vi "Begin.vi"(8 "error in":errorcluster) -> (0 "error out":errorcluster)   [LabVIEW 2017]
doc: "Called before other user functions, this VI is expected to open initial I/O refnums, load in file data, and do all program initialization. Notice that the <B>error out</B> terminal is simply used for data flow. Wiring it to other structures or subVIs ensures that this VI runs first."
uses:
  <vilib>/Rock Robotics/WPI/DriverStation/WPI_DriverStationRobotMode2.ctl
  <vilib>/Rock Robotics/WPI/Joystick/WPI_JoystickDeviceEnum.ctl
  <vilib>/Rock Robotics/SystemInterfaces/DIO/FPGA_DIOPWMChannel.ctl
  <vilib>/Rock Robotics/WPI/Solenoid/WPI_SolenoidChannel.ctl
  <vilib>/Rock Robotics/WPI/ThirdParty/Cross The Road Electronics/Phoenix-LabVIEW/Motor Controller/Controls/CTRE_Phoenix_MotorControl_ControlMode.ctl
  <vilib>/Rock Robotics/WPI/SafetyOutput/WPI_SafetyOutputConfigMenu.ctl
  <vilib>/Rock Robotics/WPI/ThirdParty/Cross The Road Electronics/Phoenix-LabVIEW/Motor Controller/Controls/CTRE_Phoenix_MotorControl_LimitSwitchSource_Local.ctl
  <vilib>/Rock Robotics/WPI/ThirdParty/Cross The Road Electronics/Phoenix-LabVIEW/Motor Controller/Controls/CTRE_Phoenix_MotorControl_LimitSwitchNormal.ctl
  Robot Global Data.vi
  <vilib>/Rock Robotics/Network Tables/NT Write String Array.vi
  <vilib>/Rock Robotics/Network Tables/NT Write String.vi
  5492_OrientationButtonPress.vi
  5492_DriveOrientation.vi
  5492_SpitButton.vi
  5492_LiftButtons.vi
  5492_DriveRamp.vi
  <vilib>/Rock Robotics/WPI/Solenoid/WPI_SolenoidOpenDouble.vi
  5492_SlowButton.vi
  5492_InitialYaw.vi
  5492_CollectButtons.vi
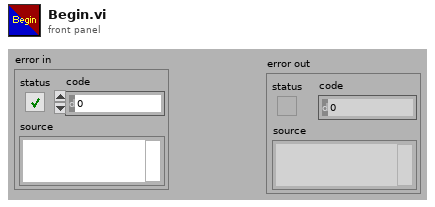
[diagram p1: front panel]
types:
  T1 = typedef "WPI_SafetyOutputConfigMenu.ctl" = enum16{"Enable", "Disable"}
  T2 = typedef "FPGA_DIOPWMChannel.ctl" = enum8{"PWM 0", "PWM 1", "PWM 2", "PWM 3", "PWM 4", "PWM 5", "PWM 6", "PWM 7", "PWM 8", "PWM 9", "PWM MXP 0", "PWM MXP 1", "PWM MXP 2", "PWM MXP 3", "PWM MXP 4", "PWM MXP 5", "PWM MXP 6", "PWM MXP 7", "PWM MXP 8", "PWM MXP 9", "Invalid"}
  T3 = typedef "CTRE_Phoenix_MotorControl_ControlMode.ctl" = u16
  T4 = typedef "CTRE_Phoenix_MotorControl_LimitSwitchNormal.ctl" = enum16{"Normally Open", "Normally Closed", "Disabled"}
  T5 = typedef "CTRE_Phoenix_MotorControl_LimitSwitchSource_Local.ctl" = enum16{"Feedback Connector", "Remote Talon SRX", "Remote CANifier", "Deactivated"}
  T6 = typedef "WPI_SolenoidChannel.ctl" = enum8{"Solenoid 0", "Solenoid 1", "Solenoid 2", "Solenoid 3", "Solenoid 4", "Solenoid 5", "Solenoid 6", "Solenoid 7", "Invalid"}
  T7 = typedef "WPI_JoystickDeviceEnum.ctl" = enum16{"USB 0", "USB 1", "USB 2", "USB 3", "USB 4", "USB 5"}
  T8 = typedef "WPI_DriverStationRobotMode2.ctl" = enum16{"Autonomous Disabled", "Autonomous Enabled", "Teleop Disabled", "Teleop Enabled", "Disconnected", "Finish", "Test Disabled", "Test Enabled", "Emergency Stopped"}
  T9 = typedef "WPI_JoystickDevRef.ctl" = cluster{"Device":T7}
  T10 = typedef "WPI_RobotDriveDevRef.ctl" = cluster{"DevStatus":errorcluster, "Motors[]":T11[], "Square Inputs":bool, "Max Output":dbl}
  T11 = typedef "WPI_MotorControlDeviceRef.ctl" = cluster{"DeviceStatus":errorcluster, "Type":T12, "PWM":cluster{"PWM Channel":T2, "DeadBand":T13}, "CAN":cluster{"Device Number":u8, "SetOutput VI Ref":variant, "GetOutput VI Ref":variant, "Enable VI Ref":variant, "Disable VI Ref":variant, "Data":variant}, "Invert":bool, "DIO PWM":cluster{"PWM \"Enable\" Channel":T2, "DIOChannel":T14, "PWM Rate":dbl}}
  T12 = typedef "WPI_MotorControlType.ctl" = enum16{"PWM", "CAN", "DIO PWM"}
  T13 = typedef "WPI_PWMDeadband.ctl" = cluster{"Name":string, "maxPositivePwm":i32, "minPositivePwm":i32, "centerPwm":i32, "maxNegativePwm":i32, "minNegativePwm":i32, "angularRange":u16}
  T14 = typedef "FPGA_DIOChannel.ctl" = enum8{"DIO 0", "DIO 1", "DIO 2", "DIO 3", "DIO 4", "DIO 5", "DIO 6", "DIO 7", "DIO 8", "DIO 9", "DIO MXP 0", "DIO MXP 1", "DIO MXP 2", "DIO MXP 3", "DIO MXP 4", "DIO MXP 5", "DIO MXP 6", "DIO MXP 7", "DIO MXP 8", "DIO MXP 9", "DIO MXP 10", "DIO MXP 11", "DIO MXP 12", "DIO MXP 13", "DIO MXP 14", "DIO MXP 15", "SPI Port CS1", "SPI Port CS2", "SPI Port CS3", "SPI Port MISO", "SPI Port MOSI", "Invalid"}
  T15 = typedef "WPI_SolenoidDevRef.ctl" = cluster{"DevStatus":errorcluster, "Pneumatics Control Module":u8, "Forward Solenoid Channel":T6, "Reverse Solenoid Channel":T6}
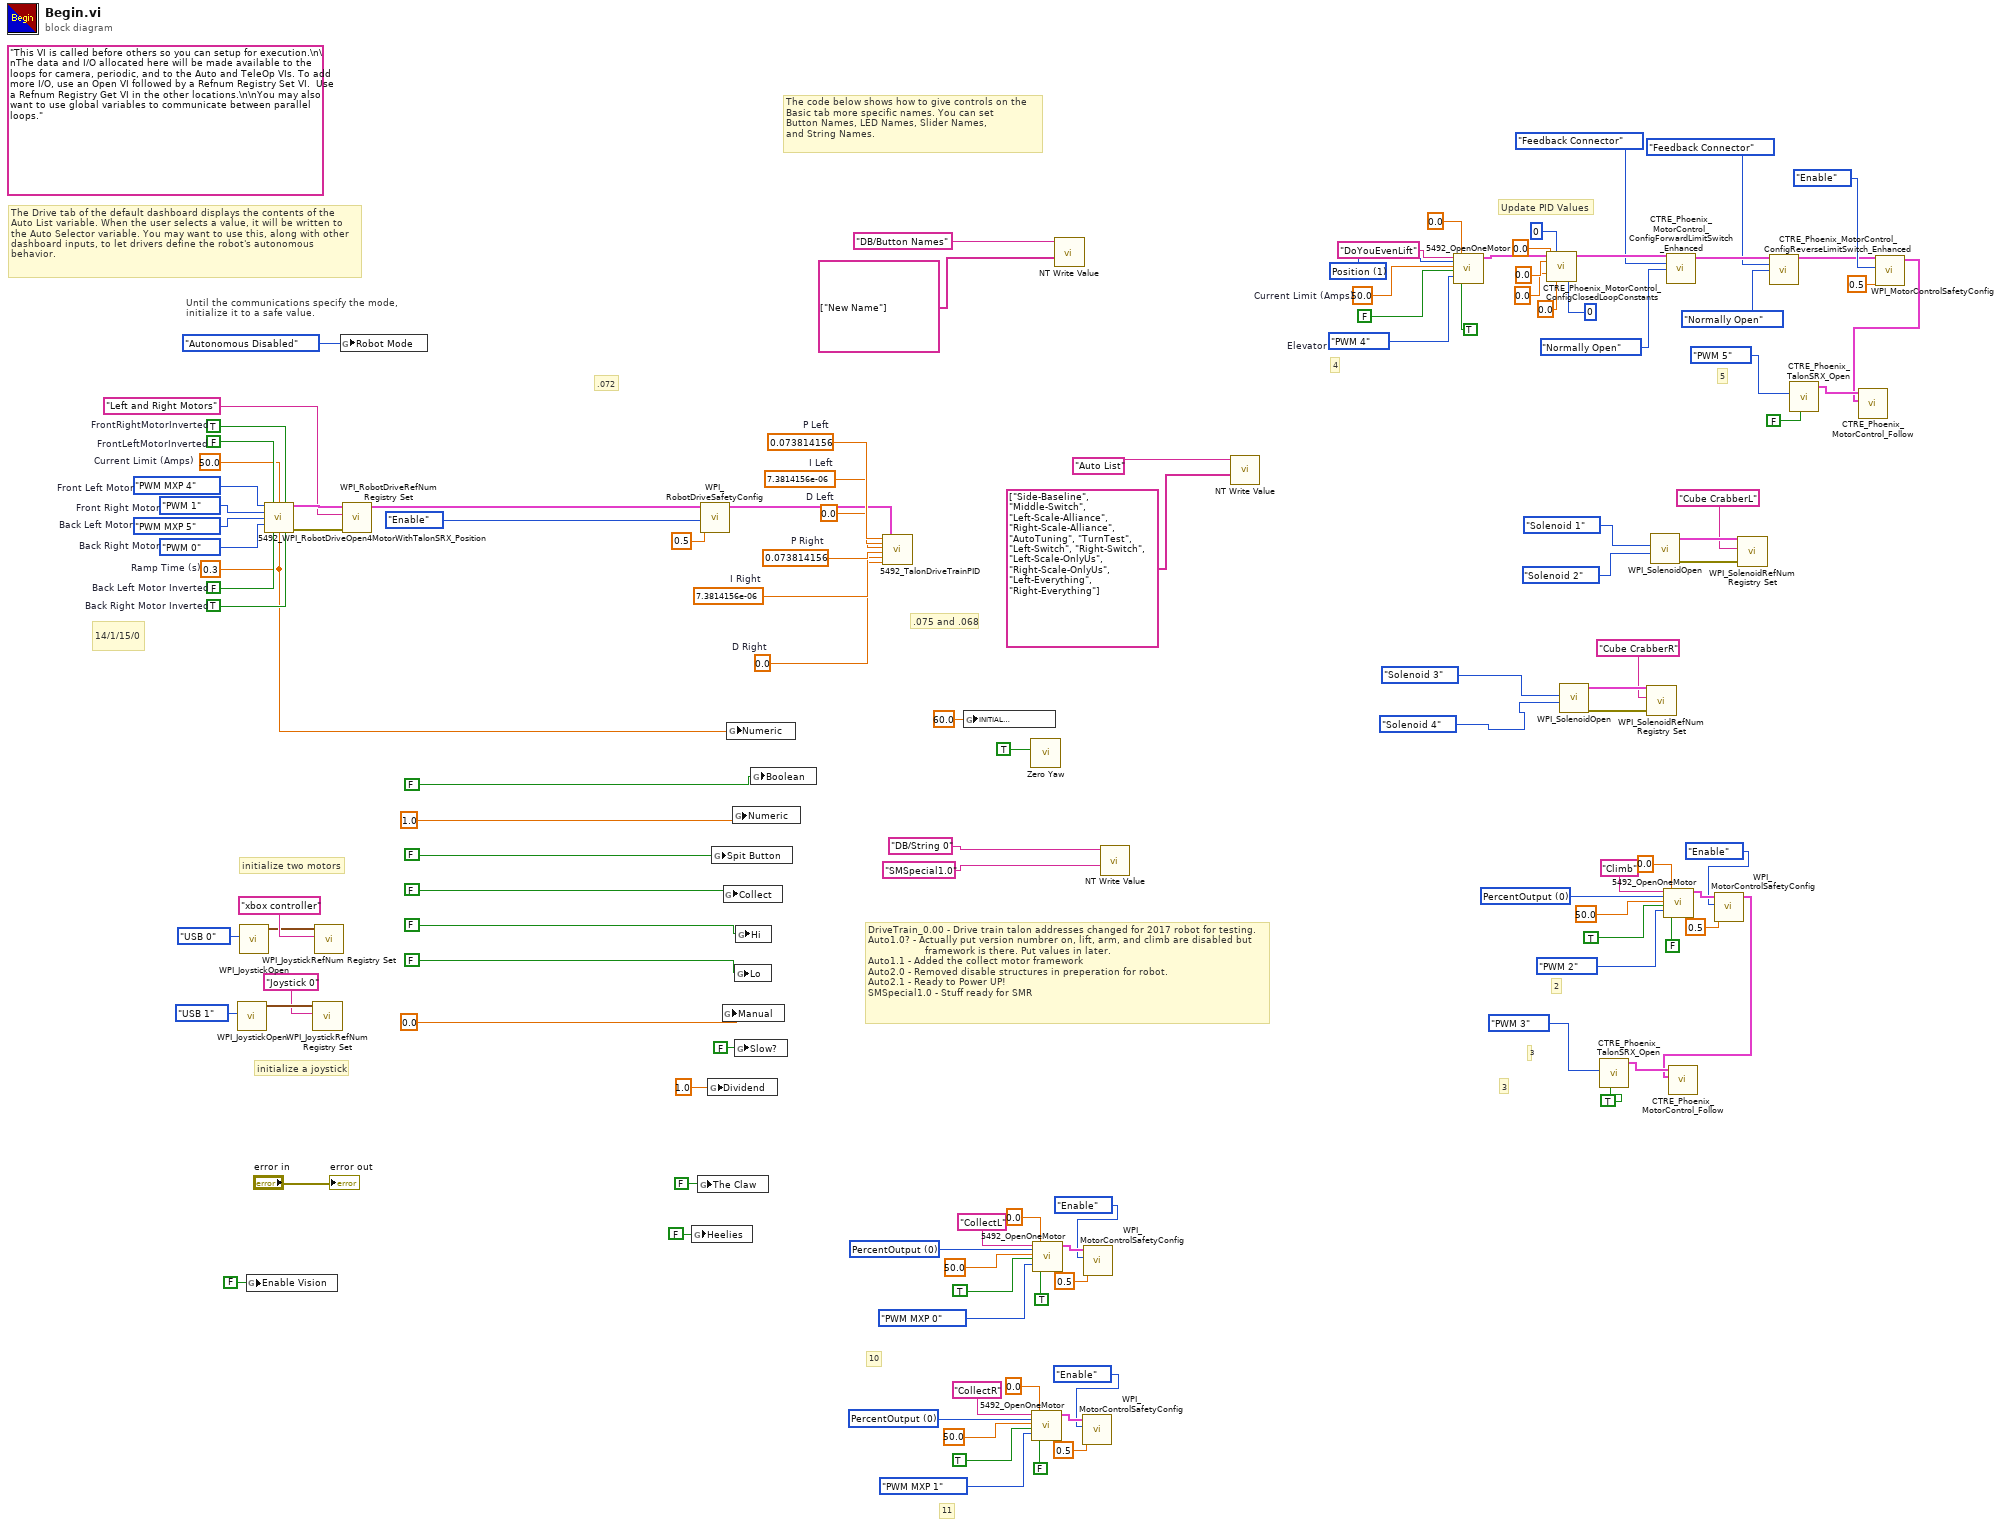
[diagram p0: block diagram]
diagram:
  w3 = T3 0 items=["PercentOutput"=0, "Position"=1, "Velocity"=2, "Current"=3, "Follower"=5, "MotionProfile"=6, "MotionMagic"=7, "MotionMagicArc"=8, "MotionProfileArc"=10, "Disabled"=15] ("Control Mode")
  w19 = T3 0 items=["PercentOutput"=0, "Position"=1, "Velocity"=2, "Current"=3, "Follower"=5, "MotionProfile"=6, "MotionMagic"=7, "MotionMagicArc"=8, "MotionProfileArc"=10, "Disabled"=15] ("Control Mode")
  w33 = T3 0 items=["PercentOutput"=0, "Position"=1, "Velocity"=2, "Current"=3, "Follower"=5, "MotionProfile"=6, "MotionMagic"=7, "MotionMagicArc"=8, "MotionProfileArc"=10, "Disabled"=15] ("Control Mode")
  w57 = FPGA_DIOPWMChannel."PWM 4"  # Elevator
  w59 = 50.0  # Current Limit (Amps)
  w60 = T3 1 items=["PercentOutput"=0, "Position"=1, "Velocity"=2, "Current"=3, "Follower"=5, "MotionProfile"=6, "MotionMagic"=7, "MotionMagicArc"=8, "MotionProfileArc"=10, "Disabled"=15] ("Control Mode")
  w81 = 0.0  # D Right
  w82 = 7.3814156e-06  # I Right
  w83 = 0.073814156  # P Right
  w84 = 0.0  # D Left
  w85 = 7.3814156e-06  # I Left
  w86 = 0.073814156  # P Left
  w65 = 0.3  # Ramp Time (s)
  w88 = 50.0  # Current Limit (Amps)
  w89 = TRUE  # Back Right Motor Inverted
  w90 = FALSE  # Back Left Motor Inverted
  w91 = FPGA_DIOPWMChannel."PWM 0"  # Back Right Motor
  w92 = FPGA_DIOPWMChannel."PWM MXP 5"  # Back Left Motor
  w95 = FPGA_DIOPWMChannel."PWM 1"  # Front Right Motor
  w96 = FPGA_DIOPWMChannel."PWM MXP 4"  # Front Left Motor
  w100 = FALSE  # FrontLeftMotorInverted
  w101 = TRUE  # FrontRightMotorInverted
  (unwired) "This VI is called before others so you can setup for execution.\n\nThe data and I/O allocated here will be made available to the loops for camera, periodic, and to the Auto and TeleOp VIs. To add more I/O, use an Open VI followed by a Refnum Registry Set VI.  Use a Refnum Registry Get VI in the other locations.\n\nYou may also want to use global variables to communicate between parallel loops."
  # ".072"
  # "11"
  # "10"
  # "3"
  # "3"
  # "2"
  # "5"
  # "Update PID Values"
  # "4"
  # ".075 and .068"
  # "14/1/15/0"
  # "DriveTrain_0.00 - Drive train talon addresses changed for 2017 robot for testing.\nAuto1.0? - Actually put version numbrer on, lift, arm, and climb are disabled but\n                   framework is there. Put values in later. \nAuto1.1 - Added the collect motor framework\nAuto2.0 - Removed disable structures in preperation for robot.\nAuto2.1 - Ready to Power UP!\nSMSpecial1.0 - Stuff ready for SMR"
  # "The Drive tab of the default dashboard displays the contents of the\nAuto List variable. When the user selects a value, it will be written to\nthe Auto Selector variable. You may want to use this, along with other\ndashboard inputs, to let drivers define the robot's autonomous\nbehavior."
  # "The code below shows how to give controls on the\nBasic tab more specific names. You can set\nButton Names, LED Names, Slider Names,\nand String Names."
  # "initialize a joystick"
  # "Until the communications specify the mode,\ninitialize it to a safe value."
  # "initialize two motors"
  n1 = call <vilib>:"WPI_JoystickOpen.vi"("JoystickDevice"=WPI_JoystickDeviceEnum."USB 1") -> ("JoystickDevRef"=w108:T9)  [unwired: 10 in]
  n2 = call <vilib>:"WPI_JoystickOpen.vi"("JoystickDevice"=WPI_JoystickDeviceEnum."USB 0") -> ("JoystickDevRef"=w120:T9)  [unwired: 10 in]
  n3 = global write "Robot Global Data.vi" "Enable Vision"(FALSE ("Enable Vision")) -> ()
  n4 = call "5492_WPI_RobotDriveOpen4MotorWithTalonSRX_Position.vi"("Front Left Motor"=w96, "Front Left Motor Inverted"=w100, "Current Limit (Amps)"=w88, "Front Right Motor Inverted"=w101, "Front Right Motor"=w95, "Back Left Motor"=w92, "Back Right Motor"=w91, "Back Left Motor Inverted"=w90, "Ramp Time (s)"=w65, "Back Right Motor Inverted"=w89) -> ("RobotDriveDevRef"=w99:T10, "error out"=w97:errorcluster)  [unwired: 4 in]
  n5 = call <vilib>:"WPI_JoystickRefNum Registry Set.vi"("refnum name"="Joystick 0", "JoystickDevRef"=w108) -> ()  [unwired: 8 in, 2 out]
  n6 = call <vilib>:"WPI_JoystickRefNum Registry Set.vi"("refnum name"="xbox controller", "JoystickDevRef"=w120) -> ()  [unwired: 8 in, 2 out]
  n7 = global write "Robot Global Data.vi" "Robot Mode"(WPI_DriverStationRobotMode2."Autonomous Disabled" ("Robot Mode")) -> ()
  n8 = call <vilib>:"WPI_RobotDriveRefNum Registry Set.vi"("error in (no error)"=w97, "refnum name"="Left and Right Motors", "RobotDriveDevRef"=w99) -> ("RobotDriveDevRef"=w94:T10)  [unwired: 1 in, 7 out]
  n9 = global write "5492_CollectButtons.vi" "Heelies"(FALSE ("Heelies")) -> ()
  n10 = global write "5492_CollectButtons.vi" "The Claw"(FALSE ("The Claw")) -> ()
  n11 = call <vilib>:"WPI_RobotDriveSafetyConfig.vi"("timeout (s)"=0.5, "mode"=WPI_SafetyOutputConfigMenu."Enable", "RobotDriveDevRef"=w94) -> ("RobotDriveDevRef"=w80:T10)  [unwired: 7 in, 1 out]
  n12 = global write "5492_SlowButton.vi" "Dividend"(1.0 ("Dividend")) -> ()
  n13 = global write "5492_SpitButton.vi" "Spit Button"(FALSE) -> ()
  n14 = global write "5492_LiftButtons.vi" "Manual"(0.0 ("Manual")) -> ()
  n15 = global write "5492_LiftButtons.vi" "Collect"(FALSE ("Collect")) -> ()
  n16 = global write "5492_DriveRamp.vi" "Numeric"(w65) -> ()
  n17 = global write "5492_DriveOrientation.vi" "Numeric"(1.0 ("Numeric")) -> ()
  n18 = global write "5492_LiftButtons.vi" "Lo"(FALSE ("Collect")) -> ()
  n19 = global write "5492_SlowButton.vi" "Slow?"(FALSE ("Slow?")) -> ()
  n20 = global write "5492_LiftButtons.vi" "Hi"(FALSE ("Collect")) -> ()
  n21 = global write "5492_OrientationButtonPress.vi" "Boolean"(FALSE ("Boolean")) -> ()
  n22 = call "5492_TalonDriveTrainPID.vi"("P Left"=w86, "I Left"=w85, "D Left"=w84, "P Right"=w83, "I Right"=w82, "D Right"=w81, "RobotDriveDevRef 2"=w80) -> ()  [unwired: 12 in, 1 out]
  n23 = global write "5492_InitialYaw.vi" "INITIAL\n YAW"(60.0 ("INITIAL\n YAW")) -> ()
  n24 = call <vilib>:"Zero Yaw.vi"("Zero"=TRUE) -> ()  [unwired: 11 in]
  n25 = call "5492_OpenOneMotor.vi"("refnum name"="CollectR", "Control Mode"=w3, "Current Limit (Amps)"=50.0, "Current Limit?"=TRUE, "Device Number"=FPGA_DIOPWMChannel."PWM MXP 1", "Output"=0.0, "Invert"=FALSE) -> ("MotorControlDevRef"=w9:T11)  [unwired: 11 in, 1 out]
  n26 = call "5492_OpenOneMotor.vi"("refnum name"="CollectL", "Control Mode"=w19, "Current Limit (Amps)"=50.0, "Current Limit?"=TRUE, "Device Number"=FPGA_DIOPWMChannel."PWM MXP 0", "Output"=0.0, "Invert"=TRUE) -> ("MotorControlDevRef"=w13:T11)  [unwired: 11 in, 1 out]
  n27 = call-poly <vilib>:"NT Write Value.vi"("String Array"=string[] ["New Name"], "Name"="DB/Button Names") -> ()  [unwired: 9 in, 1 out]
  n28 = call <vilib>:"WPI_MotorControlSafetyConfig.vi"("timeout (s)"=0.5, "mode"=WPI_SafetyOutputConfigMenu."Enable", "MotorControlDevRef"=w9) -> ()  [unwired: 7 in, 2 out]
  n29 = call <vilib>:"WPI_MotorControlSafetyConfig.vi"("timeout (s)"=0.5, "mode"=WPI_SafetyOutputConfigMenu."Enable", "MotorControlDevRef"=w13) -> ()  [unwired: 7 in, 2 out]
  n30 = call-poly <vilib>:"NT Write Value.vi"("String"="SMSpecial1.0", "Name"="DB/String 0") -> ()  [unwired: 9 in, 1 out]
  n31 = call-poly <vilib>:"NT Write Value.vi"("String Array"=string[] ["Side-Baseline", "Middle-Switch", "Left-Scale-Alliance", "Right-Scale-Alliance", "AutoTuning", "TurnTest", "Left-Switch", "Right-Switch", "Left-Scale-OnlyUs", "Right-Scale-OnlyUs", "Left-Everything", "Right-Everything"], "Name"="Auto List") -> ()  [unwired: 9 in, 1 out]
  n32 = call "5492_OpenOneMotor.vi"("refnum name"="DoYouEvenLift", "Control Mode"=w60, "Current Limit (Amps)"=w59, "Current Limit?"=FALSE, "Device Number"=w57, "Output"=0.0, "Invert"=TRUE) -> ("MotorControlDevRef"=w54:T11)  [unwired: 11 in, 1 out]
  n33 = call <vilib>:"CTRE_Phoenix_MotorControl_ConfigClosedLoopConstants.vi"("PhoenixMotorControlDevRef"=w54, "slotIdx"=0, "P"=0.0, "I"=0.0, "D"=0.0, "F"=0.0, "timeoutMs"=0) -> ("PhoenixMotorControlDevRef"=w45:T11)  [unwired: 7 in, 1 out]
  n34 = call-poly <vilib>:"WPI_SolenoidOpen.vi"("Reverse Solenoid Channel"=WPI_SolenoidChannel."Solenoid 4", "Forward Solenoid Channel"=WPI_SolenoidChannel."Solenoid 3") -> ("error out"=w70:errorcluster, "SolenoidDevRef"=w69:T15)  [unwired: 8 in]
  n35 = call <vilib>:"CTRE_Phoenix_TalonSRX_Open.vi"("Invert"=TRUE, "Device Number"=FPGA_DIOPWMChannel."PWM 3") -> ("CAN Talon SRX Ref"=w24:T11)  [unwired: 8 in, 1 out]
  n36 = call <vilib>:"WPI_SolenoidRefNum Registry Set.vi"("error in (no error)"=w70, "refnum name"="Cube CrabberR", "SolenoidDevRef"=w69) -> ()  [unwired: 7 in, 2 out]
  n37 = call-poly <vilib>:"WPI_SolenoidOpen.vi"("Reverse Solenoid Channel"=WPI_SolenoidChannel."Solenoid 2", "Forward Solenoid Channel"=WPI_SolenoidChannel."Solenoid 1") -> ("error out"=w79:errorcluster, "SolenoidDevRef"=w78:T15)  [unwired: 8 in]
  n38 = call "5492_OpenOneMotor.vi"("refnum name"="Climb", "Control Mode"=w33, "Current Limit (Amps)"=50.0, "Current Limit?"=TRUE, "Device Number"=FPGA_DIOPWMChannel."PWM 2", "Output"=0.0, "Invert"=FALSE) -> ("MotorControlDevRef"=w27:T11)  [unwired: 11 in, 1 out]
  n39 = call <vilib>:"CTRE_Phoenix_MotorControl_ConfigForwardLimitSwitch_Enhanced.vi"("PhoenixMotorControlDevRef"=w45, "Limit Switch Source"=CTRE_Phoenix_MotorControl_LimitSwitchSource_Local."Feedback Connector", "NormallyOpenOrClosed"=CTRE_Phoenix_MotorControl_LimitSwitchNormal."Normally Open") -> ("PhoenixMotorControlDevRef"=w44:T11)  [unwired: 11 in, 1 out]
  n40 = call <vilib>:"WPI_MotorControlSafetyConfig.vi"("timeout (s)"=0.5, "mode"=WPI_SafetyOutputConfigMenu."Enable", "MotorControlDevRef"=w27) -> ("MotorControlDevRef"=w22:T11)  [unwired: 7 in, 1 out]
  n41 = call <vilib>:"CTRE_Phoenix_MotorControl_Follow.vi"("Master Controller to Follow"=w22, "PhoenixMotorControlDevRef"=w24) -> ()  [unwired: 8 in, 2 out]
  n42 = call <vilib>:"WPI_SolenoidRefNum Registry Set.vi"("error in (no error)"=w79, "refnum name"="Cube CrabberL", "SolenoidDevRef"=w78) -> ()  [unwired: 7 in, 2 out]
  n43 = call <vilib>:"CTRE_Phoenix_MotorControl_ConfigReverseLimitSwitch_Enhanced.vi"("PhoenixMotorControlDevRef"=w44, "Limit Switch Source"=CTRE_Phoenix_MotorControl_LimitSwitchSource_Local."Feedback Connector", "NormallyOpenOrClosed"=CTRE_Phoenix_MotorControl_LimitSwitchNormal."Normally Open") -> ("PhoenixMotorControlDevRef"=w43:T11)  [unwired: 11 in, 1 out]
  n44 = call <vilib>:"CTRE_Phoenix_TalonSRX_Open.vi"("Invert"=FALSE, "Device Number"=FPGA_DIOPWMChannel."PWM 5") -> ("CAN Talon SRX Ref"=w38:T11)  [unwired: 8 in, 1 out]
  n45 = call <vilib>:"WPI_MotorControlSafetyConfig.vi"("timeout (s)"=0.5, "mode"=WPI_SafetyOutputConfigMenu."Enable", "MotorControlDevRef"=w43) -> ("MotorControlDevRef"=w36:T11)  [unwired: 7 in, 1 out]
  n46 = call <vilib>:"CTRE_Phoenix_MotorControl_Follow.vi"("Master Controller to Follow"=w36, "PhoenixMotorControlDevRef"=w38) -> ()  [unwired: 8 in, 2 out]
  "error out" <- "error in"
